vi "P1.vi"(1 "N2":dbl, 2 "N1":dbl) -> (0 "NO":dbl)   [LabVIEW 2010]
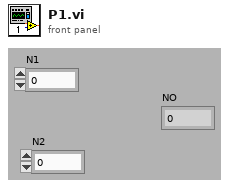
[diagram p1: front panel]
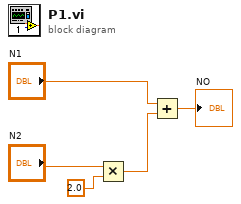
[diagram p0: block diagram]
diagram:
  n1 = Multiply(x="N2", y=2.0) -> (x*y=w2:dbl)
  n2 = Add(x="N1", y=w2) -> (x+y=→"NO":dbl)
